vi "rql_Create gRPC Client.vi"(4 "Show in Debugger?":bool=TRUE, 6 "Message Priority":T1=enum."Normal", 8 "error in":errorcluster, 10 "Data in":T2, 11 "gRPC Client Tester in":refnum<class "gRPC Client Tester.lvclass">) -> (0 "error out":errorcluster, 3 "dup gRPC Client Tester out":refnum<class "gRPC Client Tester.lvclass">)   [LabVIEW 2019, in "gRPC Client Tester.lvclass"]
doc: "This VI sends a <b>Local API Request</b> message to an MHL case of the Worker that owns this VI.\n---\nCreates the bidi gRPC Client and begins connection to the Server."
uses:
  gRPC Client Tester.lvclass
  <vilib>/addons/_Workers/Library/Case Label.ctl
  <vilib>/addons/_Workers/Library/Workers.lvlib
  <vilib>/addons/_Workers/Library/Classes/Message/Priority.ctl
  <vilib>/addons/_Workers/Library/Classes/Message/Message.lvclass
  rql_Create gRPC Client.ctl
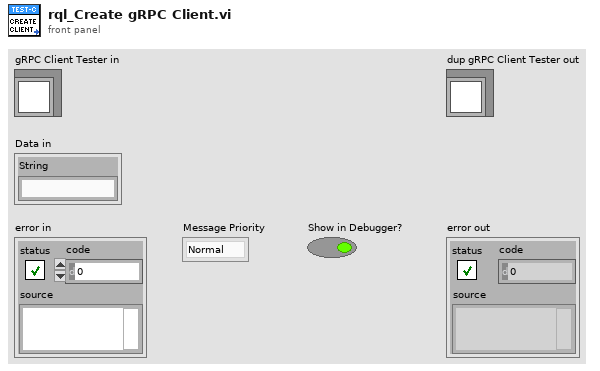
[diagram p1: front panel]
types:
  T1 = typedef "Workers.lvlib/Message.lvclass/Priority.ctl" = enum16{"Low", "Normal", "High"}
  T2 = typedef "gRPC Client Tester.lvclass/rql_Create gRPC Client.ctl" = cluster{"String":string}
  T3 = typedef "Workers.lvlib/Case Label.ctl" = string
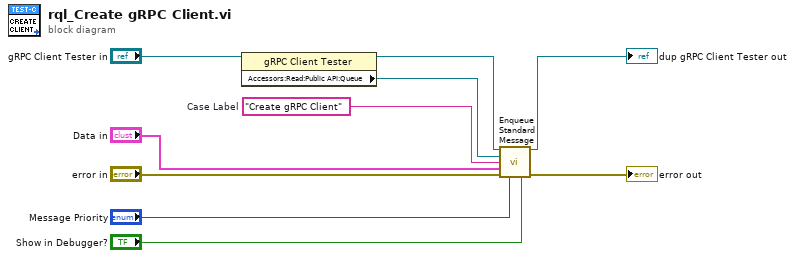
[diagram p0: block diagram]
diagram:
  w1 = T3 "Create gRPC Client"  # Case Label
  n1 = property class="gRPC Client Tester"(reference="gRPC Client Tester in") -> (reference out=w3:refnum<class "gRPC Client Tester.lvclass">, "Accessors:Read:Public API:Queue"=w2:refnum<class "Message Queue.lvclass">)  [unwired: 1 in, 1 out]
  n2 = call-dynamic "Enqueue Standard Message.vi"("Worker"=w3, "Message Queue"=w2, "Case Label"=w1, "Data"="Data in", "error in (no error)"="error in", "Priority (Normal)"="Message Priority", "Send Message to Debugger? (T)"="Show in Debugger?") -> ("dup Worker out"=→"dup gRPC Client Tester out":refnum<class "gRPC Client Tester.lvclass">, "error out"=→"error out":errorcluster)  [unwired: 7 in]
